vi "仪器时间 (子VI).vi"(4 "秒":u16, 6 "分":u16, 7 "年":u16, 9 "时":u16, 10 "日":u16, 11 "月":u16) -> (3 "time stamp":timestamp)   [LabVIEW 2016, in "德润超标留样.lvlib"]
uses:
  <vilib>/Utility/miscctls.llb/LVDateTimeRec.ctl
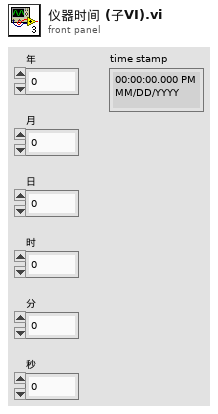
[diagram p1: front panel]
types:
  T1 = typedef "LVDateTimeRec.ctl" = cluster{"fractional second":dbl, "second":i32, "minute":i32, "hour":i32, "day of month":i32, "month":i32, "year":i32, "day of week":i32, "day of year":i32, "DST":i32}
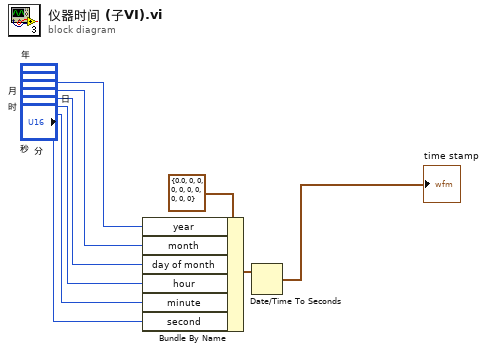
[diagram p0: block diagram]
diagram:
  n1 = Bundle By Name(cluster=T1 {"fractional second"=0.0, "second"=0, "minute"=0, "hour"=0, "day of month"=0, "month"=0, "year"=0, "day of week"=0, "day of year"=0, "DST"=0} ("日期时间记录"), "year"="年", "month"="月", "day of month"="日", "hour"="时", "minute"="分", "second"="秒") -> (w2:T1)
  n2 = Date/Time To Seconds(2:w2) -> (0:→"time stamp":timestamp)  [unwired: 1 in]
